vi "Read (Orientation Update Matrix).vi"(0 "VISA resource name":refnum<visa-resource-name>, 11 "error in (no error)":errorcluster) -> (2 "Checksum Pass":bool, 3 "Timer":u32, 4 "VISA resource name out":refnum<visa-resource-name>, 8 "Orientation Update Matrix":sgl[][](array[numeric]), 15 "error out":errorcluster)   [LabVIEW 2012, in "MicroStrain 3DM-GXx.lvlib"]
doc: "Read the Orientation Update Matrix. This is a 9 component coordinate transformation matrix which describes the change in orientation of the device during the period of the most recent calculation cycle."
uses:
  <instrlib>/MicroStrain 3DM-GXx/MicroStrain 3DM-GXx.lvlib
  <instrlib>/MicroStrain 3DM-GXx/Public/Data/Parse Message VIs/Parse (Orientation Update Matrix).vi
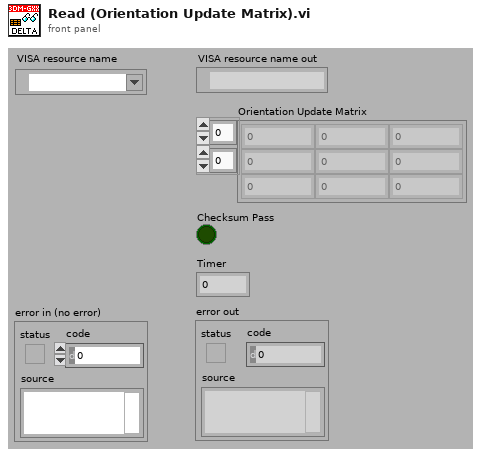
[diagram p1: front panel]
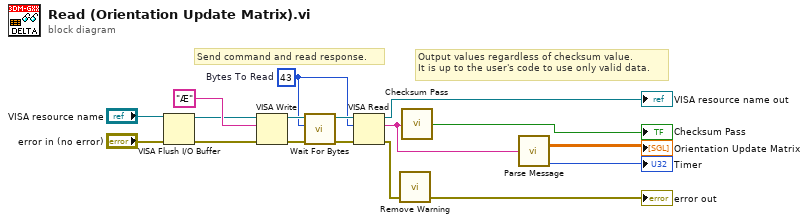
[diagram p0: block diagram]
diagram:
  w12 = u32 43  # Bytes To Read
  # "Output values regardless of checksum value.\nIt is up to the user's code to use only valid data."
  # "Send command and read response."
  n1 = VISA Flush I/O Buffer(VISA resource name="VISA resource name", error in (no error)="error in (no error)") -> (VISA resource name out=w2:refnum<visa-resource-name>, error out=w1:errorcluster)  [unwired: 1 in]
  n2 = VISA Write(VISA resource name=w2, write buffer="Æ", error in (no error)=w1) -> (VISA resource name out=w16:refnum<visa-resource-name>, error out=w15:errorcluster)  [unwired: 1 out]
  n3 = call <instrlib>:"Wait For Bytes.vi"("error in (no error)"=w15, "Bytes To Read (0)"=w12, "VISA resource name"=w16) -> ("error out"=w14:errorcluster, "VISA resource name out"=w13:refnum<visa-resource-name>)  [unwired: 7 in]
  n4 = VISA Read(VISA resource name=w13, byte count=w12, error in (no error)=w14) -> (VISA resource name out=→"VISA resource name out":refnum<visa-resource-name>, read buffer=w11:string, error out=w8:errorcluster)  [unwired: 1 out]
  n5 = call <instrlib>:"Remove Warning.vi"("error in (no error)"=w8) -> ("error out"=→"error out":errorcluster)  [unwired: 3 in, 1 out]
  n6 = call <instrlib>:"Checksum Pass.vi"("Message In"=w11) -> ("Checksum Pass"=→"Checksum Pass":bool)  [unwired: 4 in]
  n7 = call-poly <instrlib>:"Parse Message.vi"("Message In"=w11) -> ("Orientation Update Matrix"=→"Orientation Update Matrix":sgl[][], "Timer"=→"Timer":u32)  [unwired: 13 in]
